vi "pulse_generator_multiheater_refnum.vi"(2 "Stop! Refnum":refnum<vi>, 3 "Pulse Generator Control Multiheater Refnums":T1) -> ()   [LabVIEW 2017]
uses:
  pulse_generator_controls_multiheater_refnums.ctl
  <vilib>/Utility/error.llb/DialogType.ctl
  <vilib>/DAQmx/write.llb/DAQmx Write (Digital 1D Bool NChan 1Samp 1Line).vi
  <vilib>/DAQmx/write.llb/DAQmx Write (Digital Bool 1Line 1Point).vi
  <vilib>/DAQmx/create/channels.llb/DAQmx Create Channel (DO-Digital Output).vi
  <vilib>/DAQmx/create/channels.llb/DAQmx Create Channel (CO-Pulse Generation-Frequency).vi
  <vilib>/DAQmx/configure/timing.llb/DAQmx Timing (Implicit).vi
  <vilib>/DAQmx/miscellaneous.llb/DAQmx Fill In Error Info.vi
panel:
  out "Stopped!":bool caption="OK"
  in  "Stop! Local":bool
  out "message":string=" INSTRUCTIONS:\r\rNormal Use:  When using subVIs that incorporate the error in/error out (or error I/O) structure, place this handler where you want to inform the user of an error, typically at the end of the I/O data path, as the last action of the program.  If the error in error? is ERROR, the handler creates a message describing the error and its source.  If the type of dialog = 1 (default), the message is displayed to the user, who can only acknowedge it.  If the type = 2, the user can acknowledge the message or abort execution; aborting a program with active I/O is not recommended.  If the type = 0, no message is displayed; this is used to process the error programmatically, and the error out cluster elements are wired to individual terminals for that reason.  \r\rOther Use:\n\r\nlocal testing.  To test the error code of a subVI or function that does not have the error I/O structure, you can wire its error code and a source string to the local error code and error source inputs.  If error in error? indicates no error and error code is not equal to 0, the local code and source are substituted for the error in values, and error? is set TRUE (ERROR)."
  in  "SwitchHelper":bool
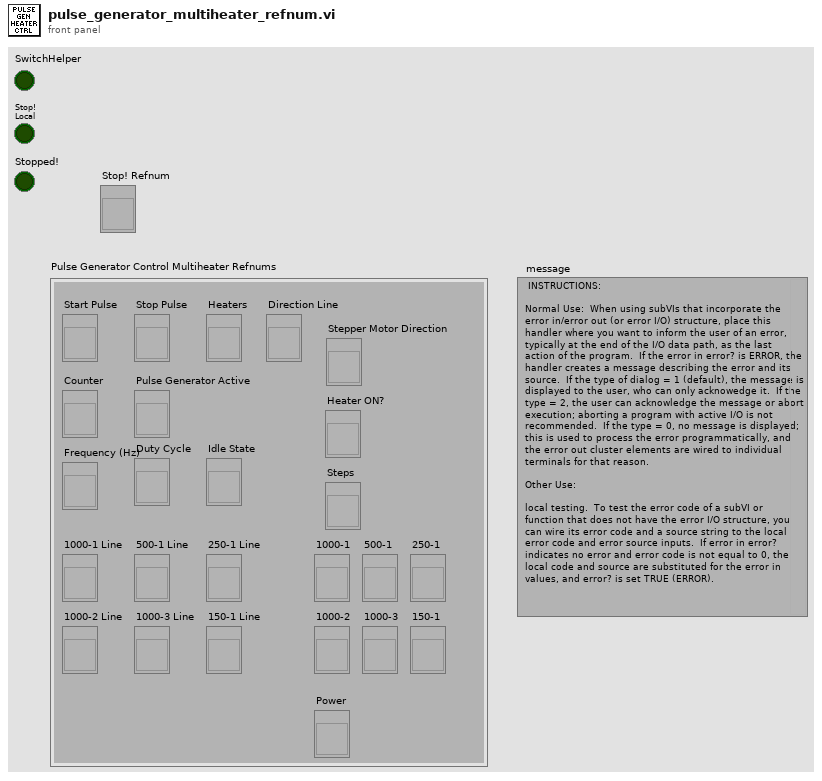
[diagram p1: front panel]
types:
  T1 = typedef "pulse_generator_controls_multiheater_refnums.ctl" = cluster{"Start Pulse":refnum<vi>, "Stop Pulse":refnum<vi>, "Heaters":refnum<vi>, "Counter":refnum<vi>, "Frequency (Hz)":refnum<vi>, "Duty Cycle":refnum<vi>, "Idle State":refnum<vi>, "Pulse Generator Active":refnum<vi>, "Stepper Motor Direction":refnum<vi>, "Steps":refnum<vi>, "Direction Line":refnum<vi>, "1000-1 Line":refnum<vi>, "1000-2 Line":refnum<vi>, "1000-3 Line":refnum<vi>, "500-1 Line":refnum<vi>, "250-1 Line":refnum<vi>, "1000-1":refnum<vi>, "1000-2":refnum<vi>, "1000-3":refnum<vi>, "500-1":refnum<vi>, "250-1":refnum<vi>, "150-1":refnum<vi>, "Heater ON?":refnum<vi>, "150-1 Line":refnum<vi>, "Power":refnum<vi>}
  T2 = enum8{"Enabled", "Disabled", "Disabled and Grayed Out"}
  T3 = typedef "DialogType.ctl" = u16
  T4 = cluster{"1000-1":refnum<vi>, "1000-2":refnum<vi>, "1000-3":refnum<vi>, "500-1":refnum<vi>, "250-1":refnum<vi>, "150-1":refnum<vi>}
  T5 = cluster{"1000-1 Line":refnum<vi>, "1000-2 Line":refnum<vi>, "1000-3 Line":refnum<vi>, "500-1 Line":refnum<vi>, "250-1 Line":refnum<vi>, "150-1 Line":refnum<vi>}
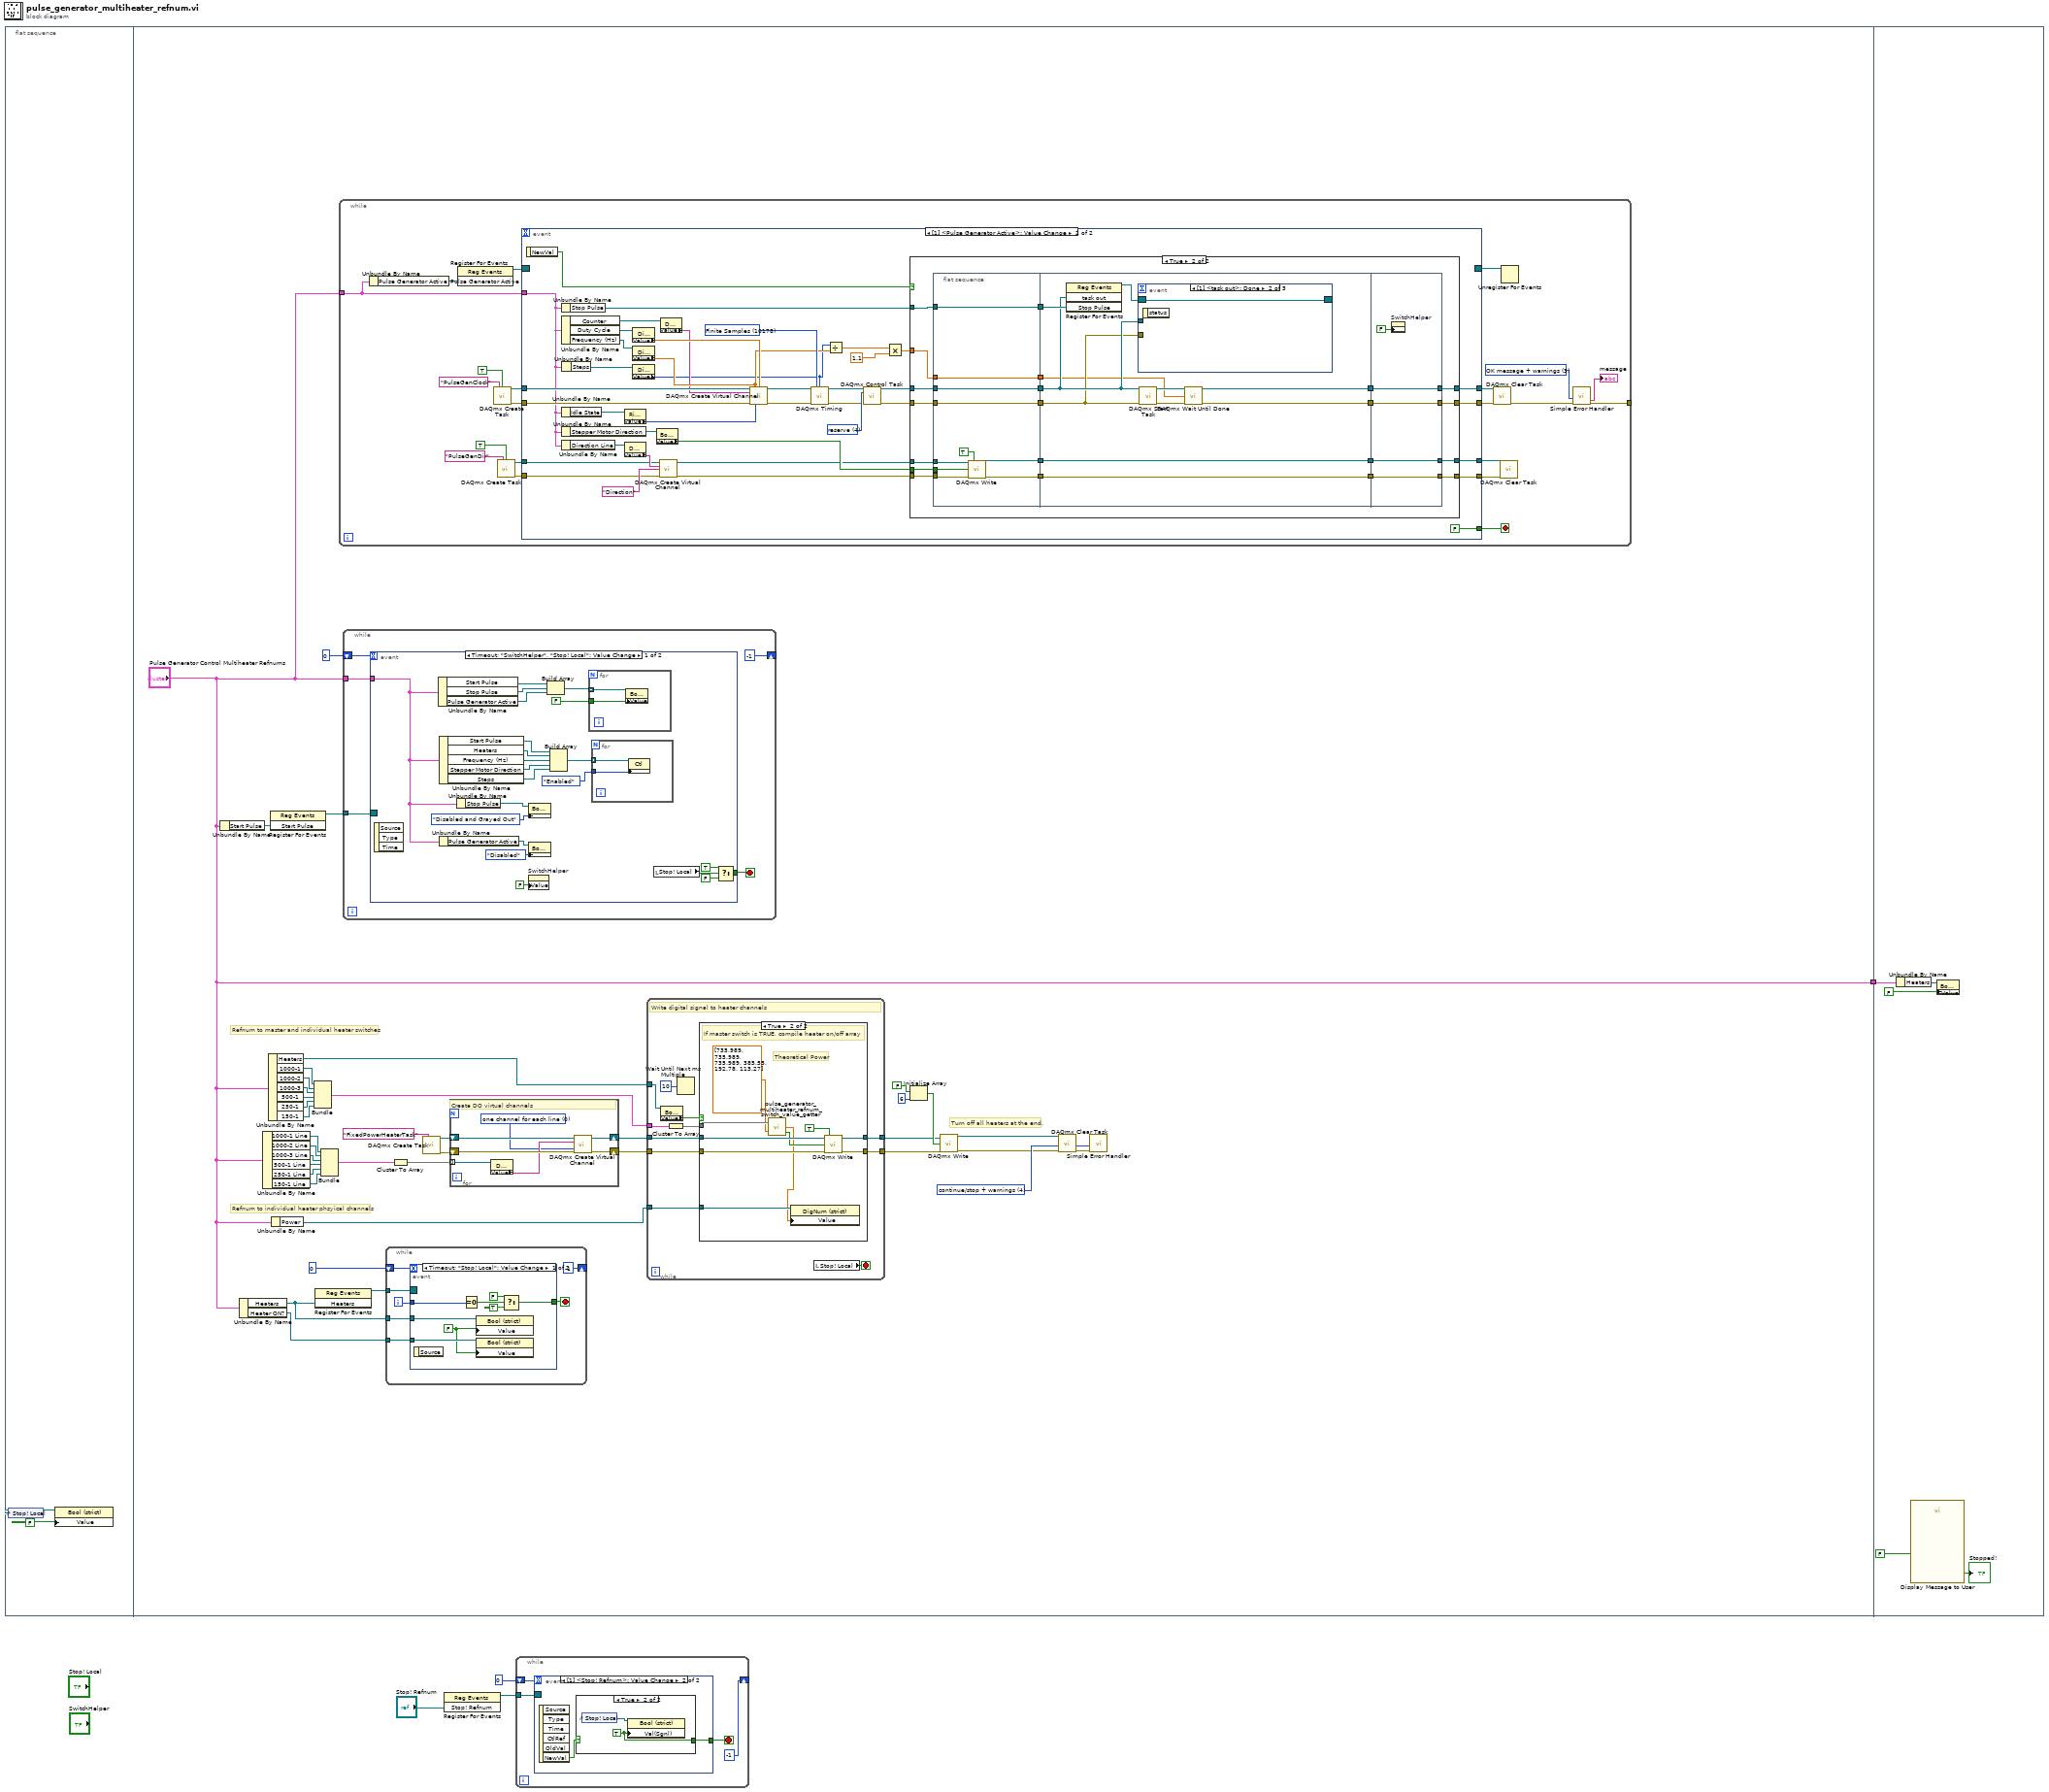
[diagram p0: block diagram]
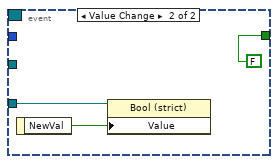
[diagram p2: hidden frame]
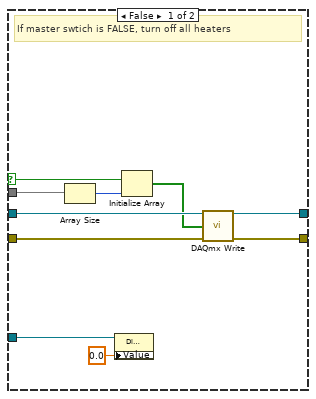
[diagram p3: hidden frame]
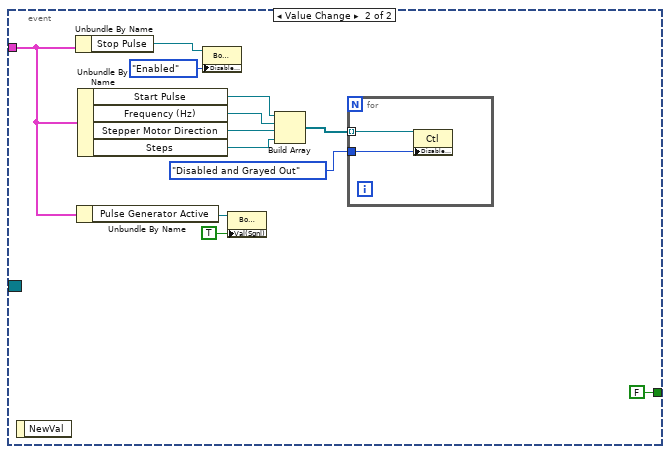
[diagram p4: hidden frame]
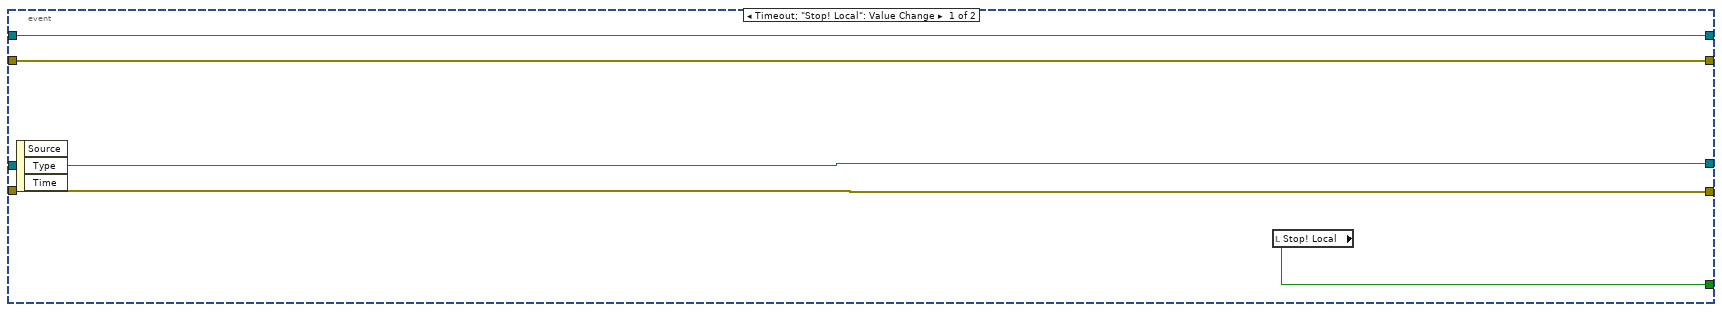
[diagram p5: hidden frame]
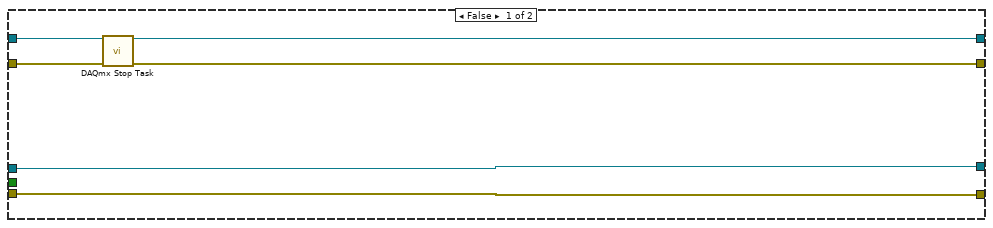
[diagram p6: hidden frame]
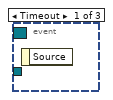
[diagram p7: hidden frame]
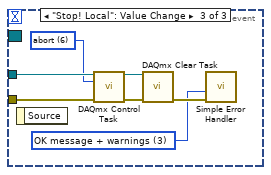
[diagram p8: hidden frame]
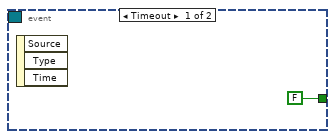
[diagram p9: hidden frame]
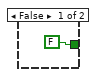
[diagram p10: hidden frame]
diagram:
  n1 = flat-sequence {
    tunnel: ["Pulse Generator Control Multiheater Refnums"] -> w1
    tunnel: w1 -> [w276]
    frame #0 {
      n2 = control-ref of="Stop! Local"() -> (w5:refnum<vi>)
      n3 = property class="Bool (strict)"(reference=w5, "Value"=FALSE) -> ()  [unwired: 1 in, 2 out]
    }
    frame #1 {
      w40 = T3 4 items=["no dialog", "OK message", "continue or stop message", "OK message + warnings", "continue/stop + warnings"] ("type of dialog (OK msg:1)")
      # "Turn off all heaters at the end."
      # "Refnum to individual heater phsyical channels"
      # "Refnum to master and individual heater switches"
      n4 = Unbundle By Name("Pulse Generator Control Multiheater Refnums") -> ("Start Pulse"=w43:refnum<vi>)
      n5 = Unbundle By Name("Pulse Generator Control Multiheater Refnums") -> ("Heaters"=w35:refnum<vi>, "Heater ON?"=w17:refnum<vi>)
      n6 = Unbundle By Name("Pulse Generator Control Multiheater Refnums") -> ("1000-1 Line"=w14:refnum<vi>, "1000-2 Line"=w13:refnum<vi>, "1000-3 Line"=w12:refnum<vi>, "500-1 Line"=w11:refnum<vi>, "250-1 Line"=w10:refnum<vi>, "150-1 Line"=w9:refnum<vi>)
      n7 = Unbundle By Name("Pulse Generator Control Multiheater Refnums") -> ("Heaters"=w34:refnum<vi>, "1000-1"=w33:refnum<vi>, "1000-2"=w32:refnum<vi>, "1000-3"=w31:refnum<vi>, "500-1"=w30:refnum<vi>, "250-1"=w28:refnum<vi>, "150-1"=w18:refnum<vi>)
      n8 = register-events(w43) -> (reference out=w44:refnum<event-registration>)  [unwired: 2 in, 1 out]
      n9 = Unbundle By Name("Pulse Generator Control Multiheater Refnums") -> ("Power"=w7:refnum<vi>)
      n10 = Bundle("1000-1"=w33, "1000-2"=w32, "1000-3"=w31, "500-1"=w30, "250-1"=w28, "150-1"=w18) -> (w15:T4)  [unwired: 1 in]
      n11 = register-events(w35) -> (reference out=w39:refnum<event-registration>)  [unwired: 2 in, 1 out]
      n12 = Bundle("1000-1 Line"=w14, "1000-2 Line"=w13, "1000-3 Line"=w12, "500-1 Line"=w11, "250-1 Line"=w10, "150-1 Line"=w9) -> (w16:T5)  [unwired: 1 in]
      n13 = while {
        tunnel: [w149] -> _
        tunnel: "Pulse Generator Control Multiheater Refnums" -> [w148]
        stop <- w159 stop-if-true
        w162 = T3 3 items=["no dialog", "OK message", "continue or stop message", "OK message + warnings", "continue/stop + warnings"] ("type of dialog (OK msg:1)")
        n14 = Unbundle By Name(w148) -> ("Pulse Generator Active"=w151:refnum<vi>)
        n15 = register-events(w151) -> (reference out=w164:refnum<event-registration>)  [unwired: 2 in, 1 out]
        n16 = call <vilib>:"DAQmx Create Task.vi"("new task name"="PulseGenClock", "auto cleanup"=TRUE) -> ("task out"=w161:refnum<k21>, "error out"=w160:errorcluster)  [unwired: 12 in]
        n17 = call <vilib>:"DAQmx Create Task.vi"("new task name"="PulseGenDir", "auto cleanup"=TRUE) -> ("task out"=w157:refnum<k21>, "error out"=w156:errorcluster)  [unwired: 12 in]
        n18 = event shown="[1] <Pulse Generator Active>: Value Change" {
          selector: w164 -> [_ _]
          dyn-events: [_ _] -> w147
          timeout: _ -> [_ _]
          tunnel: [w171 w174] -> w166
          tunnel: [w172 w173] -> w165
          tunnel: w161 -> [w172 w206]
          tunnel: w160 -> [w171 w205]
          tunnel: [w170 FALSE ("Stop! Local")] -> w159
          tunnel: w157 -> [w169 w199]
          tunnel: w156 -> [w168 w198]
          tunnel: [w169 w177] -> w150
          tunnel: [w168 w176] -> w155
          tunnel: w148 -> [_ w180]
          event Timeout; "Stop! Local": Value Change {
            n19 = event-data() -> ()  [unwired: 1 in, 3 out]
            n20 = local read "Stop! Local"() -> (w170:bool)
          }
          event Value Change {
            w195 = 4 items=["verify"=2, "reserve"=4, "commit"=3, "unreserve"=5, "abort"=6] ("action")
            w211 = 10178 items=["Finite Samples"=10178, "Continuous Samples"=10123, "Hardware Timed Single Point"=12522] ("sample mode")
            n21 = event-data() -> ("NewVal"=w212:bool)  [unwired: 1 in]
            n22 = Unbundle By Name(w180) -> ("Stop Pulse"=w186:refnum<vi>)
            n23 = Unbundle By Name(w180) -> ("Counter"=w185:refnum<vi>, "Duty Cycle"=w184:refnum<vi>, "Frequency (Hz)"=w183:refnum<vi>)
            n24 = Unbundle By Name(w180) -> ("Idle State"=w182:refnum<vi>)
            n25 = Unbundle By Name(w180) -> ("Stepper Motor Direction"=w187:refnum<vi>)
            n26 = Unbundle By Name(w180) -> ("Direction Line"=w188:refnum<vi>)
            n27 = Unbundle By Name(w180) -> ("Steps"=w179:refnum<vi>)
            n28 = property class="Ring (strict)"(reference=w182) -> ("Value"=w203:i32)  [unwired: 1 in, 2 out]
            n29 = property class="DAQmxName"(reference=w188) -> ("Value"=w202:string)  [unwired: 1 in, 2 out]
            n30 = property class="DigNum (strict)"(reference=w184) -> ("Value"=w207:dbl)  [unwired: 1 in, 2 out]
            n31 = property class="DigNum (strict)"(reference=w183) -> ("Value"=w204:dbl)  [unwired: 1 in, 2 out]
            n32 = property class="DigNum (strict)"(reference=w179) -> ("Value"=w178:i32)  [unwired: 1 in, 2 out]
            n33 = property class="Bool (strict)"(reference=w187) -> ("Value"=w200:bool)  [unwired: 1 in, 2 out]
            n34 = call-poly <vilib>:"DAQmx Create Virtual Channel.vi"("task in"=w199, "lines"=w202, "name to assign"="Direction", "error in"=w198) -> ("task out"=w190:refnum<k21>, "error out"=w189:errorcluster)  [unwired: 10 in]
            n35 = property class="DAQmxName"(reference=w185) -> ("Value"=w181:string)  [unwired: 1 in, 2 out]
            n36 = call-poly <vilib>:"DAQmx Create Virtual Channel.vi"("task in"=w206, "frequency"=w204, "duty cycle"=w207, "counter"=w181, "error in"=w205, "idle state"=w203) -> ("task out"=w197:refnum<k21>, "error out"=w196:errorcluster)  [unwired: 8 in]
            n37 = call-poly <vilib>:"DAQmx Timing.vi"("task/channels in"=w197, "sample mode"=w211, "samples per channel"=w178, "error in"=w196) -> ("task out"=w194:refnum<k21>, "error out"=w193:errorcluster)  [unwired: 10 in]
            n38 = Divide(x=w178, y=w204) -> (x/y=w209:dbl)
            n39 = call <vilib>:"DAQmx Control Task.vi"("task/channels in"=w194, "action"=w195, "error in"=w193) -> ("task out"=w191:refnum<k21>, "error out"=w192:errorcluster)  [unwired: 11 in]
            n40 = Multiply(x=w209, y=1.1) -> (x*y=w208:dbl)
            n41 = case shown="True" w212 {
              tunnel: w191 -> [w218 w236]
              tunnel: w192 -> [w217 w239]
              tunnel: [w215 w238] -> w173
              tunnel: [w216 w237] -> w174
              tunnel: w186 -> [_ w233]
              tunnel: w208 -> [_ w232]
              tunnel: w200 -> [_ w231]
              tunnel: w190 -> [w214 w230]
              tunnel: w189 -> [w213 w229]
              tunnel: [w214 w228] -> w177
              tunnel: [w213 w226] -> w176
              frame False {
                n42 = call <vilib>:"DAQmx Stop Task.vi"("task/channels in"=w218, "error in"=w217) -> ("task out"=w215:refnum<k21>, "error out"=w216:errorcluster)  [unwired: 12 in]
              }
              frame True {
                n43 = flat-sequence {
                  tunnel: w229 -> [w244]
                  tunnel: w230 -> [w245]
                  tunnel: w231 -> [w240]
                  tunnel: w232 -> [w246]
                  tunnel: w233 -> [w247]
                  tunnel: w236 -> [w248]
                  tunnel: w239 -> [w249]
                  tunnel: [w249] -> w225
                  tunnel: [w248] -> w224
                  tunnel: [w247] -> w223
                  tunnel: [w246] -> w222
                  tunnel: [w243] -> w221
                  tunnel: [w242] -> w220
                  tunnel: [w260] -> w235
                  tunnel: [w259] -> w234
                  tunnel: [w252] -> w227
                  tunnel: w225 -> [w255]
                  tunnel: w224 -> [w256]
                  tunnel: w223 -> [w257]
                  tunnel: w222 -> [w251]
                  tunnel: w221 -> [w252]
                  tunnel: w220 -> [w250]
                  tunnel: [w250] -> w219
                  tunnel: [w272] -> w237
                  tunnel: [w273] -> w238
                  tunnel: w235 -> [w273]
                  tunnel: w234 -> [w272]
                  tunnel: [w270] -> w228
                  tunnel: w227 -> [w269]
                  tunnel: [w269] -> w226
                  tunnel: w219 -> [w270]
                  frame #0 {
                    n44 = call-poly <vilib>:"DAQmx Write.vi"("task/channels in"=w245, "auto start"=TRUE, "data"=w240, "error in"=w244) -> ("task out"=w242:refnum<k21>, "error out"=w243:errorcluster)  [unwired: 9 in, 1 out]
                  }
                  frame #1 {
                    n45 = register-events(w256, w257) -> (reference out=w258:refnum<event-registration>)  [unwired: 2 in, 1 out]
                    n46 = event shown="[1] <task out>: Done" {
                      selector: w258 -> [_ w261 _]
                      dyn-events: [_ w261 _] -> _
                      timeout: _ -> [_ _ _]
                      tunnel: w256 -> [_ _ w268]
                      tunnel: w255 -> [_ _ w267]
                      event Timeout {
                        n47 = event-data() -> ()  [unwired: 1 in, 1 out]
                      }
                      event Done {
                        n48 = event-data() -> ()  [unwired: 1 in, 1 out]
                      }
                      event "Stop! Local": Value Change {
                        w262 = T3 3 items=["no dialog", "OK message", "continue or stop message", "OK message + warnings", "continue/stop + warnings"] ("type of dialog (OK msg:1)")
                        w266 = 6 items=["verify"=2, "reserve"=4, "commit"=3, "unreserve"=5, "abort"=6] ("action")
                        n49 = event-data() -> ()  [unwired: 1 in, 1 out]
                        n50 = call <vilib>:"DAQmx Control Task.vi"("task/channels in"=w268, "action"=w266, "error in"=w267) -> ("task out"=w265:refnum<k21>, "error out"=w264:errorcluster)  [unwired: 11 in]
                        n51 = call <vilib>:"DAQmx Clear Task.vi"("task in"=w265, "error in"=w264) -> ("error out"=w263:errorcluster)  [unwired: 13 in]
                        n52 = call <vilib>:"Simple Error Handler.vi"("type of dialog (OK msg:1)"=w262, "error in (no error)"=w263) -> ()  [unwired: 3 in, 5 out]
                      }
                    }
                    n53 = call <vilib>:"DAQmx Start Task.vi"("task/channels in"=w256, "error in"=w255) -> ("task out"=w254:refnum<k21>, "error out"=w253:errorcluster)  [unwired: 12 in]
                    n54 = call <vilib>:"DAQmx Wait Until Done.vi"("task/channels in"=w254, "timeout (sec)"=w251, "error in"=w253) -> ("task out"=w260:refnum<k21>, "error out"=w259:errorcluster)  [unwired: 11 in]
                  }
                  frame #2 {
                    n55 = property on="SwitchHelper" class="Bool (strict)"("Val(Sgnl)"=FALSE ("Value (Signaling)")) -> ()  [unwired: 2 in, 2 out]
                  }
                }
              }
            }
          }
        }
        n56 = call <vilib>:"DAQmx Clear Task.vi"("task in"=w165, "error in"=w166) -> ("error out"=w167:errorcluster)  [unwired: 13 in]
        n57 = call <vilib>:"DAQmx Clear Task.vi"("task in"=w150, "error in"=w155) -> ()  [unwired: 13 in, 1 out]
        n58 = Unregister For Events(event registration refnum=w147) -> ()  [unwired: 1 in, 1 out]
        n59 = call <vilib>:"Simple Error Handler.vi"("type of dialog (OK msg:1)"=w162, "error in (no error)"=w167) -> ("error out"=w149:errorcluster, "message"=→"message":string)  [unwired: 3 in, 3 out]
      }
      n60 = while {
        shift-right: [-1] -> _
        shift-left: 0 -> [w106]
        tunnel: w44 -> [w104]
        tunnel: "Pulse Generator Control Multiheater Refnums" -> [w102]
        stop <- w103 stop-if-true
        n61 = event shown="[0] Timeout;  \"SwitchHelper\", \"Stop! Local\": Value Change" {
          selector: w104 -> [_ _]
          dyn-events: _ -> [_ _]
          timeout: w106 -> [_ _]
          tunnel: [w125 FALSE ("Value")] -> w103
          tunnel: w102 -> [w107 w133]
          event Timeout; "SwitchHelper", "Stop! Local": Value Change {
            n62 = event-data() -> ()  [unwired: 1 in, 3 out]
            n63 = Unbundle By Name(w107) -> ("Start Pulse"=w114:refnum<vi>, "Stop Pulse"=w113:refnum<vi>, "Pulse Generator Active"=w112:refnum<vi>)
            n64 = Unbundle By Name(w107) -> ("Start Pulse"=w118:refnum<vi>, "Heaters"=w122:refnum<vi>, "Frequency (Hz)"=w121:refnum<vi>, "Stepper Motor Direction"=w120:refnum<vi>, "Steps"=w119:refnum<vi>)
            n65 = Unbundle By Name(w107) -> ("Pulse Generator Active"=w110:refnum<vi>)
            n66 = Unbundle By Name(w107) -> ("Stop Pulse"=w109:refnum<vi>)
            n67 = property on="SwitchHelper" class="Bool (strict)"("Value"=FALSE) -> ()  [unwired: 2 in, 2 out]
            n68 = property class="Bool (strict)"(reference=w109, "DisabledEnum"=T2."Disabled and Grayed Out" ("Disabled")) -> ()  [unwired: 1 in, 2 out]
            n69 = property class="Bool (strict)"(reference=w110, "DisabledEnum"=T2."Disabled" ("Disabled")) -> ()  [unwired: 1 in, 2 out]
            n70 = Build Array(w114, w113, w112) -> (w115:refnum<vi>[])
            n71 = Build Array(w118, w122, w121, w120, w119) -> (w117:refnum<vi>[])
            n72 = for {
              tunnel: w115 -> [w130] mode=indexing
              tunnel: FALSE ("Value") -> [w129]
              n73 = property class="Bool (strict)"(reference=w130, "Value"=w129) -> ()  [unwired: 1 in, 2 out]
            }
            n74 = for {
              tunnel: w117 -> [w132] mode=indexing
              tunnel: T2."Enabled" ("Disabled") -> [w131]
              n75 = property class="Ctl"(reference=w132, "DisabledEnum"=w131) -> ()  [unwired: 1 in, 2 out]
            }
            n76 = local read "Stop! Local"() -> (w126:bool)
            n77 = Select(t=TRUE ("Value"), s=w126, f=FALSE ("Value")) -> (s? t:f=w125:bool)
          }
          event Value Change {
            n78 = event-data() -> ()  [unwired: 1 in, 1 out]
            n79 = Unbundle By Name(w133) -> ("Stop Pulse"=w137:refnum<vi>)
            n80 = Unbundle By Name(w133) -> ("Pulse Generator Active"=w135:refnum<vi>)
            n81 = Unbundle By Name(w133) -> ("Start Pulse"=w140:refnum<vi>, "Frequency (Hz)"=w141:refnum<vi>, "Stepper Motor Direction"=w142:refnum<vi>, "Steps"=w143:refnum<vi>)
            n82 = property class="Bool (strict)"(reference=w137, "DisabledEnum"=T2."Enabled" ("Disabled")) -> ()  [unwired: 1 in, 2 out]
            n83 = property class="Bool (strict)"(reference=w135, "Val(Sgnl)"=TRUE ("Value")) -> ()  [unwired: 1 in, 2 out]
            n84 = Build Array(w140, w141, w142, w143) -> (w139:refnum<vi>[])
            n85 = for {
              tunnel: w139 -> [w146] mode=indexing
              tunnel: T2."Disabled and Grayed Out" ("Disabled") -> [w145]
              n86 = property class="Ctl"(reference=w146, "DisabledEnum"=w145) -> ()  [unwired: 1 in, 2 out]
            }
          }
        }
      }
      n87 = while {
        tunnel: w39 -> [w59]
        shift-right: [-1 ("millisecond multiple")] -> _
        shift-left: 0 ("millisecond multiple") -> [w58]
        tunnel: w35 -> [w56]
        tunnel: w17 -> [w53]
        i -> [w55]
        stop <- w54 stop-if-true
        n88 = event shown="[0] Timeout;  \"Stop! Local\": Value Change" {
          selector: w59 -> [_ _]
          dyn-events: _ -> [_ _]
          timeout: w58 -> [_ _]
          tunnel: w56 -> [w67 _]
          tunnel: w55 -> [w65 _]
          tunnel: [w62 FALSE ("f")] -> w54
          tunnel: w53 -> [w61 w68]
          event Timeout; "Stop! Local": Value Change {
            w60 = FALSE ("Value")
            n89 = event-data() -> ()  [unwired: 1 in, 1 out]
            n90 = Equal To 0?(x=w65) -> (x = 0?=w66:bool)
            n91 = property class="Bool (strict)"(reference=w67, "Value"=w60) -> ()  [unwired: 1 in, 2 out]
            n92 = property class="Bool (strict)"(reference=w61, "Value"=w60) -> ()  [unwired: 1 in, 2 out]
            n93 = Select(t=FALSE, s=w66, f=TRUE) -> (s? t:f=w62:bool)
          }
          event Value Change {
            n94 = event-data() -> ("NewVal"=w69:bool)  [unwired: 1 in]
            n95 = property class="Bool (strict)"(reference=w68, "Value"=w69) -> ()  [unwired: 1 in, 2 out]
          }
        }
      }
      n96 = Cluster To Array(cluster=w16) -> (array=w29:refnum<vi>[])
      n97 = call <vilib>:"DAQmx Create Task.vi"("new task name"="FixedPowerHeaterTask") -> ("task out"=w38:refnum<k21>, "error out"=w37:errorcluster)  [unwired: 13 in]
      n98 = for {
        tunnel: w29 -> [w48] mode=indexing
        shift-right: [w52] -> w21
        shift-left: w38 -> [w50]
        shift-right: [w51] -> w20
        shift-left: w37 -> [w49]
        w46 = 0 items=["one channel for each line", "one channel for all lines"] ("line grouping")
        # "Create DO virtual channels"
        n99 = property class="DAQmxName"(reference=w48) -> ("Value"=w47:string)  [unwired: 1 in, 2 out]
        n100 = call-poly <vilib>:"DAQmx Create Virtual Channel.vi"("task in"=w50, "lines"=w47, "line grouping"=w46, "error in"=w49) -> ("task out"=w52:refnum<k21>, "error out"=w51:errorcluster)  [unwired: 10 in]
      }
      n101 = while {
        tunnel: w21 -> [w79]
        tunnel: w20 -> [w78]
        tunnel: w34 -> [w75]
        tunnel: [w77] -> w23
        tunnel: [w76] -> w22
        tunnel: w15 -> [w73]
        tunnel: w7 -> [w71]
        stop <- w80 stop-if-true
        # "Write digital signal to heater channels"
        n102 = property class="Bool (strict)"(reference=w75) -> ("Value"=w74:bool)  [unwired: 1 in, 2 out]
        n103 = Cluster To Array(cluster=w73) -> (array=w72:refnum<vi>[])
        n104 = Wait Until Next ms Multiple(millisecond multiple=u32 10) -> ()  [unwired: 1 out]
        n105 = case shown="True" w74 {
          selector: w74 -> [w84 _]
          tunnel: w79 -> [w91 w100]
          tunnel: w78 -> [w90 w99]
          tunnel: [w88 w101] -> w77
          tunnel: [w89 w98] -> w76
          tunnel: w72 -> [w86 w96]
          tunnel: w71 -> [w83 w93]
          frame False {
            # "If master swtich is FALSE, turn off all heaters"
            n106 = Array Size(array=w86) -> (size(s)=w87:i32)
            n107 = property class="DigNum (strict)"(reference=w83, "Value"=0.0) -> ()  [unwired: 1 in, 2 out]
            n108 = Initialize Array(w84, w87) -> (w85:bool[])
            n109 = call-poly <vilib>:"DAQmx Write.vi"("task/channels in"=w91, "data"=w85, "error in"=w90) -> ("task out"=w88:refnum<k21>, "error out"=w89:errorcluster)  [unwired: 10 in, 1 out]
          }
          frame True {
            # "Theoretical Power"
            # "If master switch is TRUE, compile heater on/off array"
            n110 = call "pulse_generator_multiheater_refnum_switch_value_getter.vi"("On/Off Refnums"=w96, "Power Array"=dbl[] [735.989, 735.989, 735.989, 385.55, 192.78, 113.27]) -> ("Total Power"=w92:dbl, "Digital"=w95:bool[])  [unwired: 1 out]
            n111 = property class="DigNum (strict)"(reference=w93, "Value"=w92) -> ()  [unwired: 1 in, 2 out]
            n112 = call-poly <vilib>:"DAQmx Write.vi"("task/channels in"=w100, "auto start"=TRUE, "data"=w95, "error in"=w99) -> ("task out"=w101:refnum<k21>, "error out"=w98:errorcluster)  [unwired: 9 in, 1 out]
          }
        }
        n113 = local read "Stop! Local"() -> (w80:bool)
      }
      n114 = Initialize Array(FALSE ("element"), 6 ("dimension size")) -> (w24:bool[])
      n115 = call-poly <vilib>:"DAQmx Write.vi"("task/channels in"=w23, "data"=w24, "error in"=w22) -> ("task out"=w27:refnum<k21>, "error out"=w26:errorcluster)  [unwired: 10 in, 1 out]
      n116 = call <vilib>:"DAQmx Clear Task.vi"("task in"=w27, "error in"=w26) -> ("error out"=w42:errorcluster)  [unwired: 13 in]
      n117 = call <vilib>:"Simple Error Handler.vi"("type of dialog (OK msg:1)"=w40, "error in (no error)"=w42) -> ()  [unwired: 3 in, 5 out]
    }
    frame #2 {
      n118 = Unbundle By Name(w276) -> ("Heaters"=w275:refnum<vi>)
      n119 = call "Display Message to User"("Enable"=FALSE) -> ("OK"=→"Stopped!":bool)  [unwired: 9 in, 1 out]
      n120 = property class="Bool (strict)"(reference=w275, "Value"=FALSE) -> ()  [unwired: 1 in, 2 out]
    }
  }
  n121 = register-events("Stop! Refnum") -> (reference out=w3:refnum<event-registration>)  [unwired: 2 in, 1 out]
  n122 = while {
    tunnel: w3 -> [w282]
    shift-right: [-1] -> _
    shift-left: 0 -> [w281]
    stop <- w279 stop-if-true
    n123 = event shown="[1] <Stop! Refnum>: Value Change" {
      selector: w282 -> [_ _]
      dyn-events: _ -> [_ _]
      timeout: w281 -> [_ _]
      tunnel: [FALSE ("Value (Signaling)") w284] -> w279
      event Timeout {
        n124 = event-data() -> ()  [unwired: 1 in, 3 out]
      }
      event Value Change {
        n125 = event-data() -> ("NewVal"=w285:bool)  [unwired: 1 in, 5 out]
        n126 = case shown="True" w285 {
          tunnel: [FALSE ("Value (Signaling)") w288] -> w284
          frame False {
          }
          frame True {
            w288 = TRUE ("Value (Signaling)")
            n127 = control-ref of="Stop! Local"() -> (w287:refnum<vi>)
            n128 = property class="Bool (strict)"(reference=w287, "Val(Sgnl)"=w288) -> ()  [unwired: 1 in, 2 out]
          }
        }
      }
    }
  }
